vi "Message Handler.vi"(8 "error in (no error)":errorcluster, 11 "Zero Timeout Message Handler in":refnum<class "Zero Timeout Message Handler.lvclass">) -> (0 "error out":errorcluster, 3 "Zero Timeout Message Handler out":refnum<class "Zero Timeout Message Handler.lvclass">)   [LabVIEW 2024, in "Zero Timeout Message Handler.lvlib" / "Zero Timeout Message Handler.lvclass"]
uses:
  Zero Timeout Message Handler.lvclass
  Zero Timeout Message Handler.lvclass/Zero Timeout Message Handler.ctl
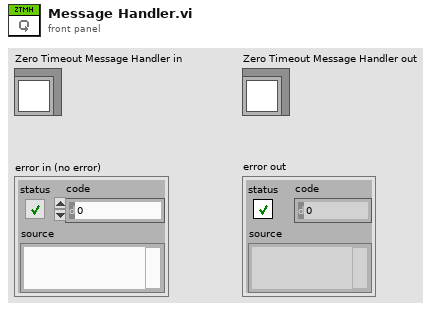
[diagram p1: front panel]
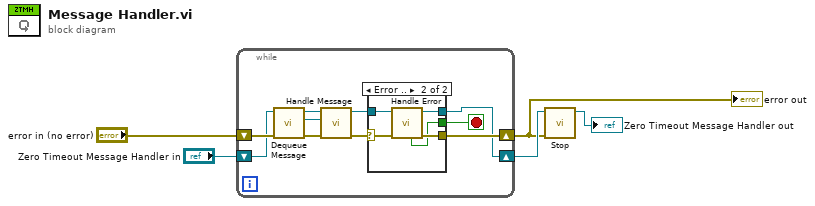
[diagram p0: block diagram]
diagram:
  n1 = while {
    shift-right: [w8] -> w1
    shift-left: "error in (no error)" -> [w14]
    shift-right: [w7] -> w4
    shift-left: "Zero Timeout Message Handler in" -> [w13]
    stop <- w6 stop-if-true
    n2 = call-dynamic "Dequeue Message.vi"("error in (no error)"=w14, "Zero Timeout Message Handler in"=w13) -> ("error out"=w15:errorcluster, "Message"=w11:refnum<class "~Message.lvclass">, "Zero Timeout Message Handler out"=w12:refnum<class "Zero Timeout Message Handler.lvclass">)  [unwired: 7 in]
    n3 = call "Handle Message.vi"("error in (no error)"=w15, "Message"=w11, "Zero Timeout Message Handler in"=w12) -> ("error out"=w10:errorcluster, "Zero Timeout Message Handler out"=w9:refnum<class "Zero Timeout Message Handler.lvclass">)  [unwired: 7 in]
    n4 = case shown="Error .." w10 {
      selector: w10 -> [w17 w18]
      tunnel: w9 -> [w16 w22]
      tunnel: [w17 w21] -> w8
      tunnel: [w16 w20] -> w7
      tunnel: [_ w19] -> w6
      frame No Error {
      }
      frame Error {
        n5 = call-dynamic "Handle Error.vi"("error in (no error)"=w18, "Zero Timeout Message Handler in"=w22) -> ("error out"=w21:errorcluster, "Zero Timeout Message Handler out"=w20:refnum<class "Zero Timeout Message Handler.lvclass">, "stop?"=w19:bool)  [unwired: 7 in]
      }
    }
  }
  "error out" <- w1
  n6 = call-dynamic "Stop.vi"("error in (no error)"=w1, "Zero Timeout Message Handler in"=w4) -> ("Zero Timeout Message Handler out"=→"Zero Timeout Message Handler out":refnum<class "Zero Timeout Message Handler.lvclass">)  [unwired: 9 in]
